vi "Asyn Rx Ch Set Protocol.vi"(9 "pstFrame":T1, 10 "Channel":u8, 11 "devId":i32) -> (1 "pstFrame out":T1, 2 "devId out":i32, 3 "function return":i32)   [LabVIEW 2013, in "CHR34XXX.lvlib"]
doc: "DLL BOOL __stdcall CHR34XXX_Asyn_Ch_Reset(IN int devId,IN BYTE Channel); DLL BOOL __stdcall CHR34XXX_Asyn_Ch_RS485LoopBack(IN int devId,IN BYTE Channel,IN BOOL Enabled); DLL BOOL __stdcall CHR34XXX_Asyn_RxCh_SetMode(IN int devId,IN BYTE Channel,IN BYTE Mode); DLL BOOL __stdcall CHR34XXX_Asyn_RxCh_SetProtocol(IN int devId,IN BYTE Channel,IN pCHRUART_ASYN_PROTOCOL_ST pstFrame);"
uses:
  CHR34XXX.lvlib
  CHR34XXX.dll
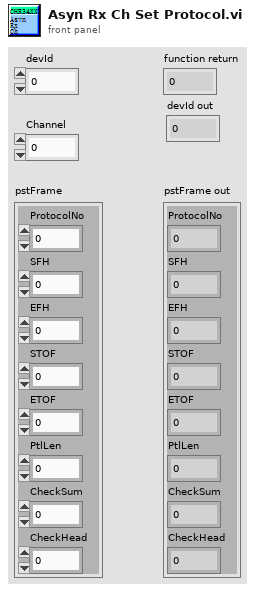
[diagram p1: front panel]
types:
  T1 = cluster{"ProtocolNo":u8, "SFH":u8, "EFH":u8, "STOF":u8, "ETOF":u8, "PtlLen":u8, "CheckSum":u8, "CheckHead":u8}
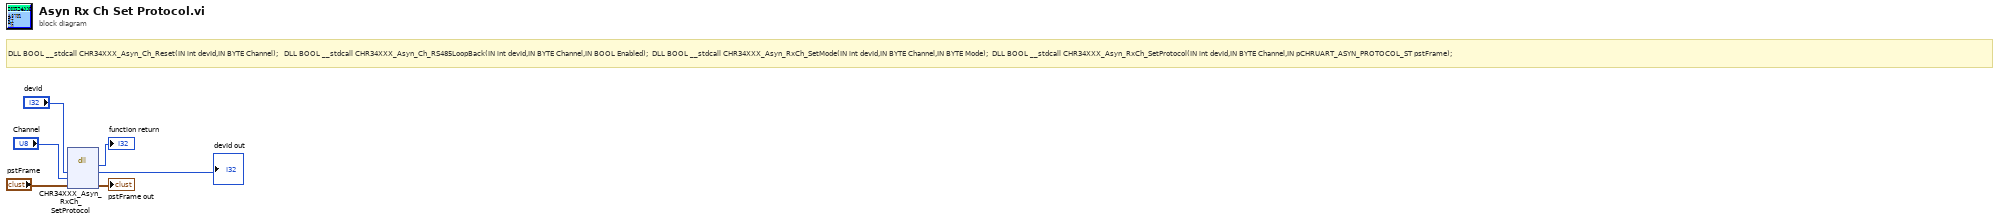
[diagram p0: block diagram]
diagram:
  # "DLL BOOL __stdcall CHR34XXX_Asyn_Ch_Reset(IN int devId,IN BYTE Channel);   DLL BOOL __stdcall CHR34XXX_Asyn_Ch_RS485LoopBack(IN int devId,IN BYTE Channel,IN BOOL Enabled);  DLL BOOL __stdcall CHR34XXX_Asyn_RxCh_SetMode(IN int devId,IN BYTE Channel,IN BYTE Mode);  DLL BOOL __stdcall CHR34XXX_Asyn_RxCh_SetProtocol(IN int devId,IN BYTE Channel,IN pCHRUART_ASYN_PROTOCOL_ST pstFrame);"
  n1 = dll-call lib="C:/Users/Administrator/Desktop/CHR34XXX_lv/lv_lib/CHR34XXX.*" fn="CHR34XXX_Asyn_RxCh_SetProtocol"("devId"="devId", "Channel"="Channel", "pstFrame"="pstFrame") -> ("返回类型"=→"function return":i32, "devId"=→"devId out":i32, "pstFrame"=→"pstFrame out":T1)  [unwired: 4 in, 2 out]
